vi "Video Power.vi"(8 "error in (no error)":errorcluster caption="错误输入（无错误）", 10 "布尔":bool, 11 "DAM0200-Relay 输入":refnum<class "DAM0200-Relay.lvclass">) -> (0 "error out":errorcluster caption="错误输出", 3 "DAM0200-Relay 输出":refnum<class "DAM0200-Relay.lvclass">)   [LabVIEW 2016, in "DAM0200-Relay.lvlib" / "DAM0200-Relay.lvclass"]
uses:
  DAM0200-Relay.lvclass
  DAM0200-Relay.lvclass/DAM0200-Relay.ctl
  <vilib>/Plasmionique/MB Master/MB Master.lvlib
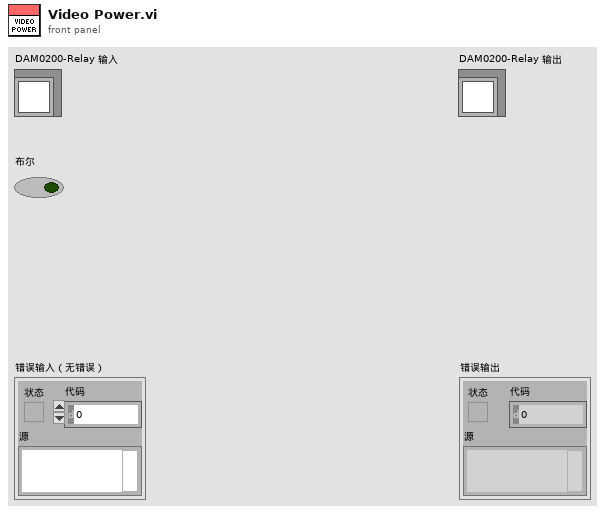
[diagram p1: front panel]
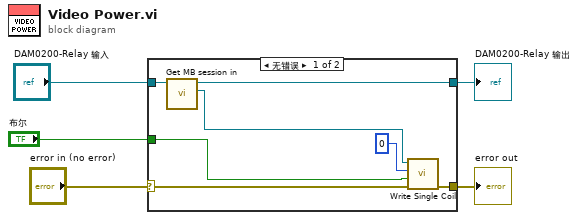
[diagram p0: block diagram]
diagram:
  n1 = case shown="无错误" "error in (no error)" {
    selector: "error in (no error)" -> [w9 w14]
    tunnel: [w8 w14] -> w4
    tunnel: [w7 w13] -> w2
    tunnel: "DAM0200-Relay 输入" -> [w12 w13]
    tunnel: "布尔" -> [w6 _]
    frame No Error {
      n2 = call "Get MB session in.vi"("DAM0200-Relay in"=w12) -> ("MB Serial Master:MB_Master"=w11:refnum<class "MB_Master.lvclass">, "DAM0200-Relay out"=w7:refnum<class "DAM0200-Relay.lvclass">)  [unwired: 9 in]
      n3 = call <vilib>:"Write Single Coil.vi"("error in (no error)"=w9, "value"=w6, "address"=u16 0, "MB session in"=w11) -> ("error out"=w8:errorcluster)  [unwired: 6 in, 1 out]
    }
    frame Error {
    }
  }
  "error out" <- w4
  "DAM0200-Relay 输出" <- w2
